vi "Pixel_Coords_to_Feature_Coords(SS).vi"(10 "Frame_Dims":sgl[](array[numeric]) min=0 max=0, 11 "Center_Coords":T1) -> (3 "Frames":T2[](array[typedef]) {"x" format="%#_4p"; "y" format="%#_4p"; "w" format="%#_4p"; "h" format="%#_4p"})   [LabVIEW 2020]
uses:
  <vilib>/Ngene/Deep Learning Toolkit/Toolkit/NN_Data/API/Data/Detection_Types/NN_BBox.ctl
  Controls/Dims(2D)ctl.ctl
  <vilib>/Ngene/Deep Learning Toolkit/Toolkit/NN_Data/API/Data/Detection_Types/NN_BBox_Format_Conversion_Direction.ctl
  <vilib>/Ngene/Deep Learning Toolkit/Toolkit/Deep_Learning_Toolkit_by_Ngene.lvlib
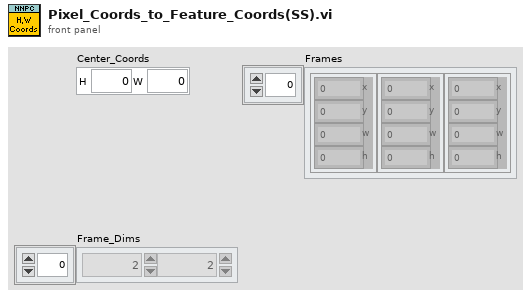
[diagram p1: front panel]
types:
  T1 = typedef "Dims(2D)ctl.ctl" = cluster{"H":i32, "W":i32}
  T2 = typedef "Deep_Learning_Toolkit_by_Ngene.lvlib/NN_BBox.ctl" = cluster{"x":sgl, "y":sgl, "w":sgl, "h":sgl}
  T3 = typedef "Deep_Learning_Toolkit_by_Ngene.lvlib/NN_BBox_Format_Conversion_Direction.ctl" = enum16{"SS_to_CWH", "CWH_to_SS"}
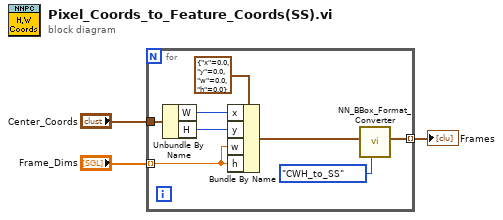
[diagram p0: block diagram]
diagram:
  n1 = for {
    tunnel: [w5] -> w3 mode=indexing
    tunnel: "Center_Coords" -> [w8]
    tunnel: "Frame_Dims" -> [w4] mode=indexing
    n2 = Unbundle By Name(w8) -> ("W"=w10:i32, "H"=w9:i32)
    n3 = Bundle By Name(cluster=T2 {"x"=0.0, "y"=0.0, "w"=0.0, "h"=0.0} ("BBox in"), "x"=w10, "y"=w9, "w"=w4, "h"=w4) -> (w6:T2)
    n4 = call <vilib>:"NN_BBox_Format_Converter.vi"("Conversion_Direction"=NN_BBox_Format_Conversion_Direction."CWH_to_SS", "BBox in"=w6) -> ("BBox out"=w5:T2)  [unwired: 9 in]
  }
  "Frames" <- w3
